vi "IL-Sensor Setting.vi"() -> (1 "IL Sensor":T1, 3 "Search Key":string)   [LabVIEW 2015]
uses:
  Galobal variable_TI.vi
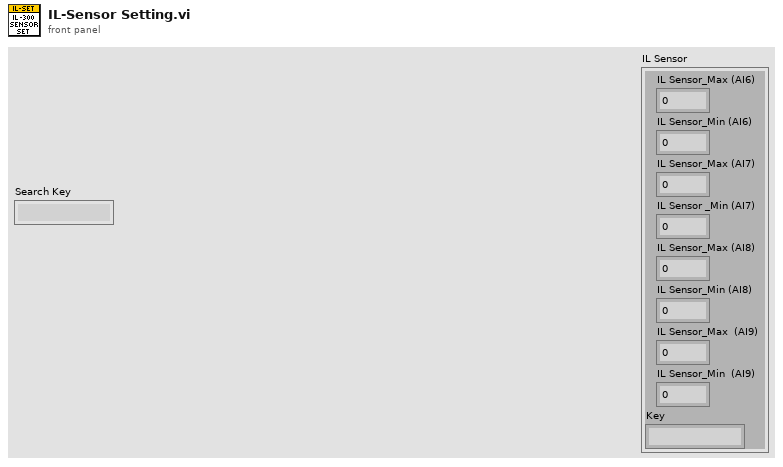
[diagram p1: front panel]
types:
  T1 = cluster{"IL Sensor_Max (AI6)":dbl, "IL Sensor_Min (AI6)":dbl, "IL Sensor_Max (AI7)":dbl, "IL Sensor _Min (AI7)":dbl, "IL Sensor_Max (AI8)":dbl, "IL Sensor_Min (AI8)":dbl, "IL Sensor_Max  (AI9)":dbl, "IL Sensor_Min  (AI9)":dbl, "Key":string}
  T2 = cluster{"IL Sensor_Max (AI6)":dbl, "IL Sensor_Min (AI6)":dbl, "IL Sensor_Max (AI7)":dbl, "IL Sensor _Min (AI7)":dbl, "IL Sensor_Max (AI8)":dbl, "IL Sensor_Min (AI8)":dbl, "IL Sensor_Max  (AI9)":dbl, "IL Sensor_Min  (AI9)":dbl}
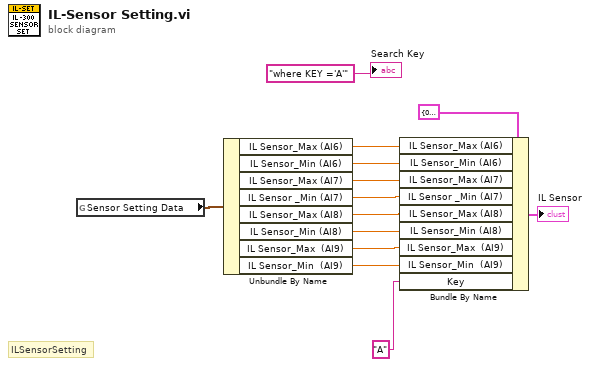
[diagram p0: block diagram]
diagram:
  # "ILSensorSetting"
  n1 = global read "Galobal variable_TI.vi" "Sensor Setting Data"() -> (w11:T2)
  n2 = Unbundle By Name(w11) -> ("IL Sensor_Max (AI6)"=w8:dbl, "IL Sensor_Min (AI6)"=w7:dbl, "IL Sensor_Max (AI7)"=w6:dbl, "IL Sensor _Min (AI7)"=w5:dbl, "IL Sensor_Max (AI8)"=w4:dbl, "IL Sensor_Min (AI8)"=w12:dbl, "IL Sensor_Max  (AI9)"=w3:dbl, "IL Sensor_Min  (AI9)"=w2:dbl)
  n3 = Bundle By Name(cluster=T1 {"IL Sensor_Max (AI6)"=0.0, "IL Sensor_Min (AI6)"=0.0, "IL Sensor_Max (AI7)"=0.0, "IL Sensor _Min (AI7)"=0.0, "IL Sensor_Max (AI8)"=0.0, "IL Sensor_Min (AI8)"=0.0, "IL Sensor_Max  (AI9)"=0.0, "IL Sensor_Min  (AI9)"=0.0, "Key"=""} ("Sensor Setting Data"), "IL Sensor_Max (AI6)"=w8, "IL Sensor_Min (AI6)"=w7, "IL Sensor_Max (AI7)"=w6, "IL Sensor _Min (AI7)"=w5, "IL Sensor_Max (AI8)"=w4, "IL Sensor_Min (AI8)"=w12, "IL Sensor_Max  (AI9)"=w3, "IL Sensor_Min  (AI9)"=w2, "Key"="A") -> (→"IL Sensor":T1)
  "Search Key" <- "where KEY ='A'"
